vi "Unwrap TCP Payload.vi"(8 "error in (no error)":errorcluster, 10 "Payload":string) -> (0 "error out":errorcluster, 2 "TcpPayload":T1)   [LabVIEW 2020, in "Vecto.lvlib"]
uses:
  Vecto.lvlib
  proto/TcpPayload/Data.ctl
  proto/TcpPayload/TcpPayload.lvlib
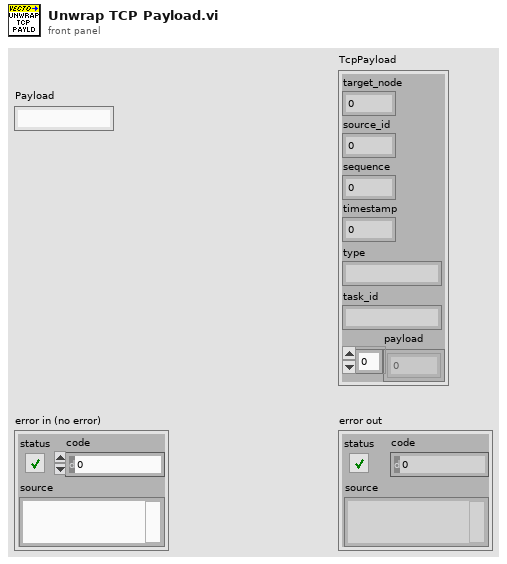
[diagram p1: front panel]
types:
  T1 = typedef "TcpPayload.lvlib/Data.ctl" = cluster{"target_node":u32, "source_id":u32, "sequence":u32, "timestamp":u64, "type":string, "task_id":string, "payload":u8[]}
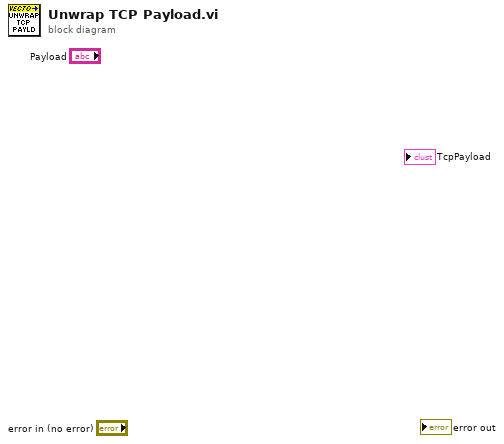
[diagram p0: block diagram]
diagram:
